vi "Set Maximum Graph Area.vi"(8 "error in (no error)":errorcluster, 11 "Waveform Chart":refnum<vi>) -> (0 "error out":errorcluster)   [LabVIEW 2021, in "IObject.lvclass"]
uses:
  IObject.lvclass
  <vilib>/Utility/miscctls.llb/LVRectTypeDef.ctl
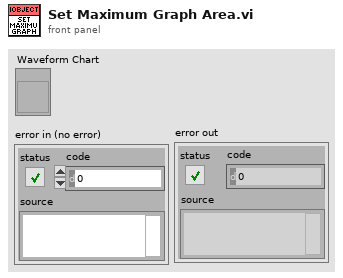
[diagram p1: front panel]
types:
  T1 = typedef "LVRectTypeDef.ctl" = cluster{"Left":i16, "Top":i16, "Right":i16, "Bottom":i16}
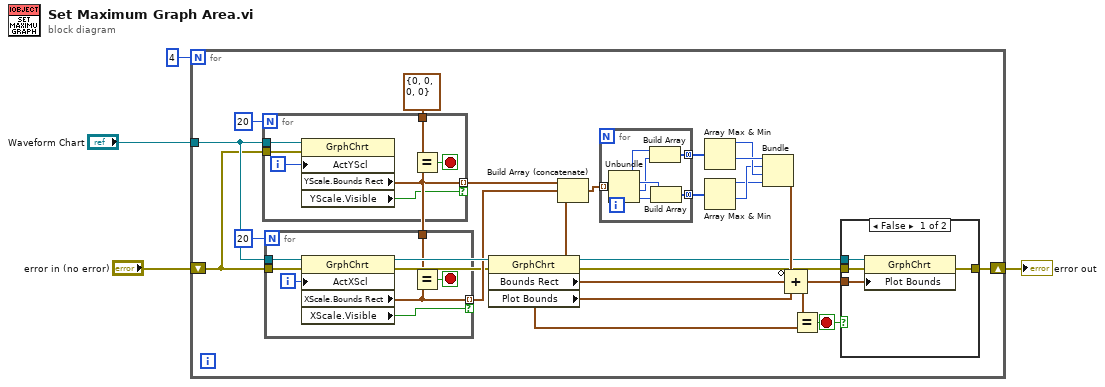
[diagram p0: block diagram]
diagram:
  n1 = for {
    N: 4 -> [_]
    tunnel: "Waveform Chart" -> [w26]
    shift-right: [w7] -> w2
    shift-left: "error in (no error)" -> [w6]
    stop <- w9 stop-if-true
    w11 = T1 {"Left"=0, "Top"=0, "Right"=0, "Bottom"=0} ("y")
    n2 = for {
      N: 20 -> [_]
      tunnel: [w50] -> w24 mode=indexing if=w52
      tunnel: w26 -> [w48]
      tunnel: w11 -> [w47]
      tunnel: w6 -> [w46]
      i -> [w51]
      stop <- w49 stop-if-true
      n3 = property on="Property Node" class="GrphChrt"(reference=w48, error in=w46, "ActYScl"=w51) -> ("YScale.Bounds Rect"=w50:T1, "YScale.Visible"=w52:bool)  [unwired: 2 out]
      n4 = Equal?(x=w47, y=w50) -> (x = y?=w49:bool)
    }
    n5 = for {
      N: 20 -> [_]
      tunnel: [w43] -> w22 mode=indexing if=w45
      tunnel: w26 -> [w41]
      tunnel: w11 -> [w40]
      tunnel: w6 -> [w39]
      i -> [w44]
      stop <- w42 stop-if-true
      n6 = property on="Property Node" class="GrphChrt"(reference=w41, error in=w39, "ActXScl"=w44) -> ("XScale.Bounds Rect"=w43:T1, "XScale.Visible"=w45:bool)  [unwired: 2 out]
      n7 = Equal?(x=w40, y=w43) -> (x = y?=w42:bool)
    }
    n8 = property on="Property Node" class="GrphChrt"(reference=w26, error in=w6) -> (reference out=w12:refnum<vi>, error out=w8:errorcluster, "Bounds Rect"=w14:T1, "Plot Bounds"=w5:T1)
    n9 = Build Array (concatenate)(w24, w22, w5) -> (w21:T1[])
    n10 = for {
      tunnel: w21 -> [w38] mode=indexing
      tunnel: [w34] -> w20 mode=concatenating
      tunnel: [w35] -> w19 mode=concatenating
      n11 = Unbundle(w38) -> ("Left"=w37:i16, "Top"=w36:i16, "Right"=w32:i16, "Bottom"=w33:i16)
      n12 = Build Array(w37, w32) -> (w34:i16[])
      n13 = Build Array(w36, w33) -> (w35:i16[])
    }
    n14 = Array Max & Min(array=w20) -> (max value=w17:i16, min value=w18:i16)  [unwired: 2 out]
    n15 = Array Max & Min(array=w19) -> (max value=w15:i16, min value=w16:i16)  [unwired: 2 out]
    n16 = Bundle(w18, w16, w17, w15) -> (w13:cluster{i16, i16, i16, i16})  [unwired: 1 in]
    n17 = Compound Arithmetic op=ADD(invert w13, w14, w5) -> (w10:T1)
    n18 = Equal?(x=w10, y=w5) -> (x = y?=w9:bool)
    n19 = case shown="False" w9 {
      tunnel: w12 -> [w30 _]
      tunnel: w10 -> [w29 _]
      tunnel: w8 -> [w28 w31]
      tunnel: [w27 w31] -> w7
      frame False {
        n20 = property on="Property Node" class="GrphChrt"(reference=w30, error in=w28, "Plot Bounds"=w29) -> (error out=w27:errorcluster)  [unwired: 1 out]
      }
      frame True {
      }
    }
  }
  "error out" <- w2
